vi "getInheritanceChain.vi"(8 "error in (no error)":errorcluster, 11 "LLNode in":refnum<class "LLNode.lvclass">) -> (0 "error out":errorcluster, 2 "Inheritance Chain":string[](array[string]), 3 "LLNode out":refnum<class "LLNode.lvclass">)   [LabVIEW 2009, in "LLNode.lvclass"]
doc: "Returns the inheritance chain."
uses:
  LLNode.lvclass
  Node/Node.lvclass
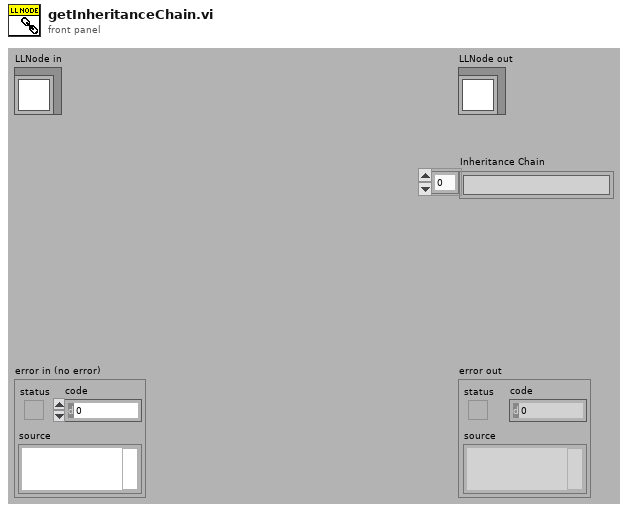
[diagram p1: front panel]
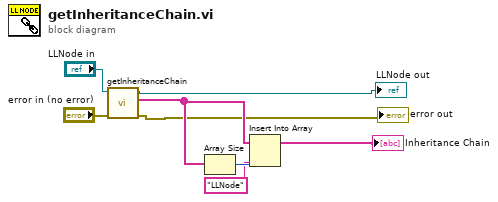
[diagram p0: block diagram]
diagram:
  n1 = call-parent "getInheritanceChain.vi"("error in (no error)"="error in (no error)", "Node in"="LLNode in") -> ("error out"=→"error out":errorcluster, "Inheritance Chain"=w4:string[], "Node out"=→"LLNode out":refnum<class "LLNode.lvclass">)  [unwired: 7 in]
  n2 = Array Size(array=w4) -> (size(s)=w6:i32)
  n3 = Insert Into Array(array=w4, index=w6, new element="LLNode") -> (→"Inheritance Chain":string[])
